vi "Close Ports 2.vi"(11 "GIC Input":T1={"     Use ?\nOff       On"=[FALSE, TRUE, FALSE, TRUE], "Mode:"=FALSE, "Rx Prop Port"="", "Hokuyo Port"="COM7", "Tx Prop  Port"="COM6", "Compass Port"="", "GPS Port"="", "Num of WPs"=0, "WP Lats and Longs"={"WP Lats"=[], "WP Longs"=[]}, "Obst Lats and Longs"={"Obst Lats"=[], "Obst Longs"=[]}, "Parameters"=[], "GPS Data"=[], "Compass"=0.0, "LMS Vector"=[], "Vision Vector"=[], "Direction Cmd"=0.0, "Speed Cmd"=0.0, "WP Vector"=[], "WP Number"=0, "Extra"=0, "SW Map"=[], "Path Cluster"={"Path x node"=[], "Path y node"=[]}} {"Obst Lats and Longs"."Obst Longs" format="%#_8g"; "Obst Lats and Longs"."Obst Lats" format="%#_8g"}) -> ()   [LabVIEW 2014]
uses:
  Hokuyo URG Series.lvlib
panel:
  # "Close Ports 2"
  # "Input:"
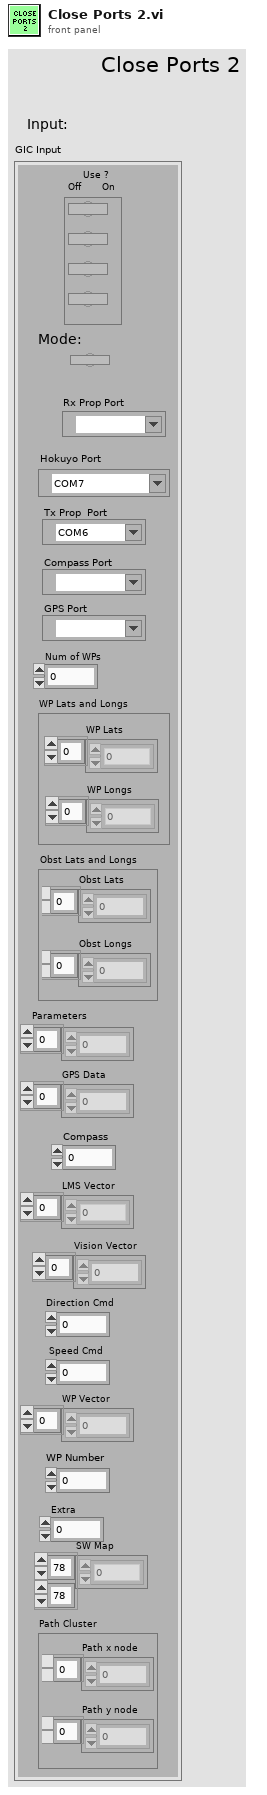
[diagram p1: front panel]
types:
  T1 = cluster{"     Use ?\nOff       On":bool[], "Mode:":bool, "Rx Prop Port":refnum<visa-resource-name>, "Hokuyo Port":refnum<visa-resource-name>, "Tx Prop  Port":refnum<visa-resource-name>, "Compass Port":refnum<visa-resource-name>, "GPS Port":refnum<visa-resource-name>, "Num of WPs":i16, "WP Lats and Longs":cluster{"WP Lats":dbl[], "WP Longs":dbl[]}, "Obst Lats and Longs":cluster{"Obst Lats":dbl[], "Obst Longs":dbl[]}, "Parameters":dbl[], "GPS Data":dbl[], "Compass":dbl, "LMS Vector":dbl[], "Vision Vector":dbl[], "Direction Cmd":dbl, "Speed Cmd":dbl, "WP Vector":dbl[], "WP Number":i32, "Extra":i16, "SW Map":i32[][], "Path Cluster":cluster{"Path x node":dbl[], "Path y node":dbl[]}}
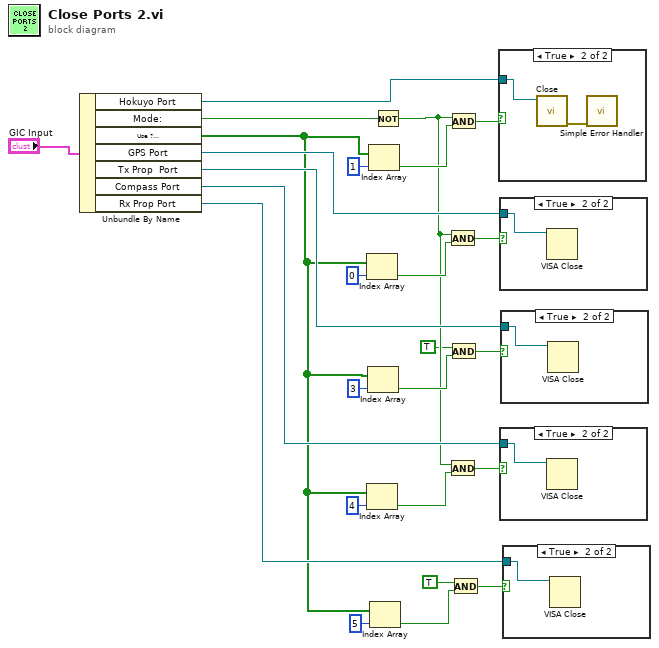
[diagram p0: block diagram]
diagram:
  n1 = Unbundle By Name("GIC Input") -> ("Hokuyo Port"=w23:refnum<visa-resource-name>, "Mode:"=w21:bool, "Use ?\nOff       On"=w5:bool[], "GPS Port"=w17:refnum<visa-resource-name>, "Tx Prop  Port"=w13:refnum<visa-resource-name>, "Compass Port"=w10:refnum<visa-resource-name>, "Rx Prop Port"=w6:refnum<visa-resource-name>)
  n2 = Index Array(array=w5, index=0) -> (element=w18:bool)
  n3 = Index Array(array=w5, index=4) -> (element=w4:bool)
  n4 = Index Array(array=w5, index=3) -> (element=w14:bool)
  n5 = Index Array(array=w5, index=1) -> (element=w25:bool)
  n6 = Index Array(array=w5, index=5) -> (element=w7:bool)
  n7 = Not(x=w21) -> (.not. x?=w3:bool)
  n8 = And(x=w3, y=w18) -> (x .and. y?=w19:bool)
  n9 = And(x=w3, y=w4) -> (x .and. y?=w11:bool)
  n10 = And(x=w3, y=w25) -> (x .and. y?=w24:bool)
  n11 = And(x=TRUE, y=w14) -> (x .and. y?=w15:bool)
  n12 = And(x=TRUE, y=w7) -> (x .and. y?=w8:bool)
  n13 = case shown="True" w24 {
    tunnel: w23 -> [_ w27]
    frame False {
    }
    frame True {
      n14 = call "Close.vi"("VISA resource name"=w27) -> ("error out"=w28:errorcluster)  [unwired: 10 in]
      n15 = call <vilib>:"Simple Error Handler.vi"("error in (no error)"=w28) -> ()  [unwired: 4 in, 5 out]
    }
  }
  n16 = case shown="True" w19 {
    tunnel: w17 -> [_ w29]
    frame False {
    }
    frame True {
      n17 = VISA Close(VISA resource name=w29) -> ()  [unwired: 1 in, 1 out]
    }
  }
  n18 = case shown="True" w11 {
    tunnel: w10 -> [_ w30]
    frame False {
    }
    frame True {
      n19 = VISA Close(VISA resource name=w30) -> ()  [unwired: 1 in, 1 out]
    }
  }
  n20 = case shown="True" w15 {
    tunnel: w13 -> [_ w31]
    frame False {
    }
    frame True {
      n21 = VISA Close(VISA resource name=w31) -> ()  [unwired: 1 in, 1 out]
    }
  }
  n22 = case shown="True" w8 {
    tunnel: w6 -> [_ w32]
    frame False {
    }
    frame True {
      n23 = VISA Close(VISA resource name=w32) -> ()  [unwired: 1 in, 1 out]
    }
  }
